vi "nana_4-ZN_O - temp.vi"() -> ()   [LabVIEW 2015]
uses:
  <vilib>/MakerHub/LINX/Public/Peripherals/Digital/Digital Write N Chans.vi
  <vilib>/MakerHub/LINX/Public/Peripherals/Analog/Analog Read 1 Chan.vi
  <vilib>/MakerHub/LINX/Private/Local IO/LinxDigitalWrite.vi
  <vilib>/MakerHub/LINX/Public/Utilities/Check Channel.vi
  <vilib>/MakerHub/LINX/Public/Peripherals/Analog/Analog Read N Chans.vi
  <vilib>/MakerHub/LINX/Private/Local IO/LinxI2cWrite.vi
  <vilib>/MakerHub/LINX/Private/Local IO/LinxAnalogRead.vi
  <vilib>/MakerHub/LINX/Public/Utilities/Open Serial.vi
  <vilib>/MakerHub/LINX/Private/Utilties/Generate Error.vi
  <vilib>/MakerHub/LINX/LMH-LINX.lvlib
panel:
  out "A1":dbl
  out "A2":dbl
  in  "T(V)":dbl
  in  "time post":u32
  in  "number of pulses":i32
  in  "low delay":u32
  in  "peak delay":u32
  out "Ref":dbl(graph)
  in  "LED":refnum<visa-resource-name>="N/A"
  out "3":dbl(graph)
  out "2":dbl(graph)
  out "4":dbl(graph)
  out "1":dbl(graph)
  out "pos":dbl
  in  "milliseconds to wait":u32
  in  "time pre":u32
  in  "Serial Port Analog":refnum<visa-resource-name>="N/A"
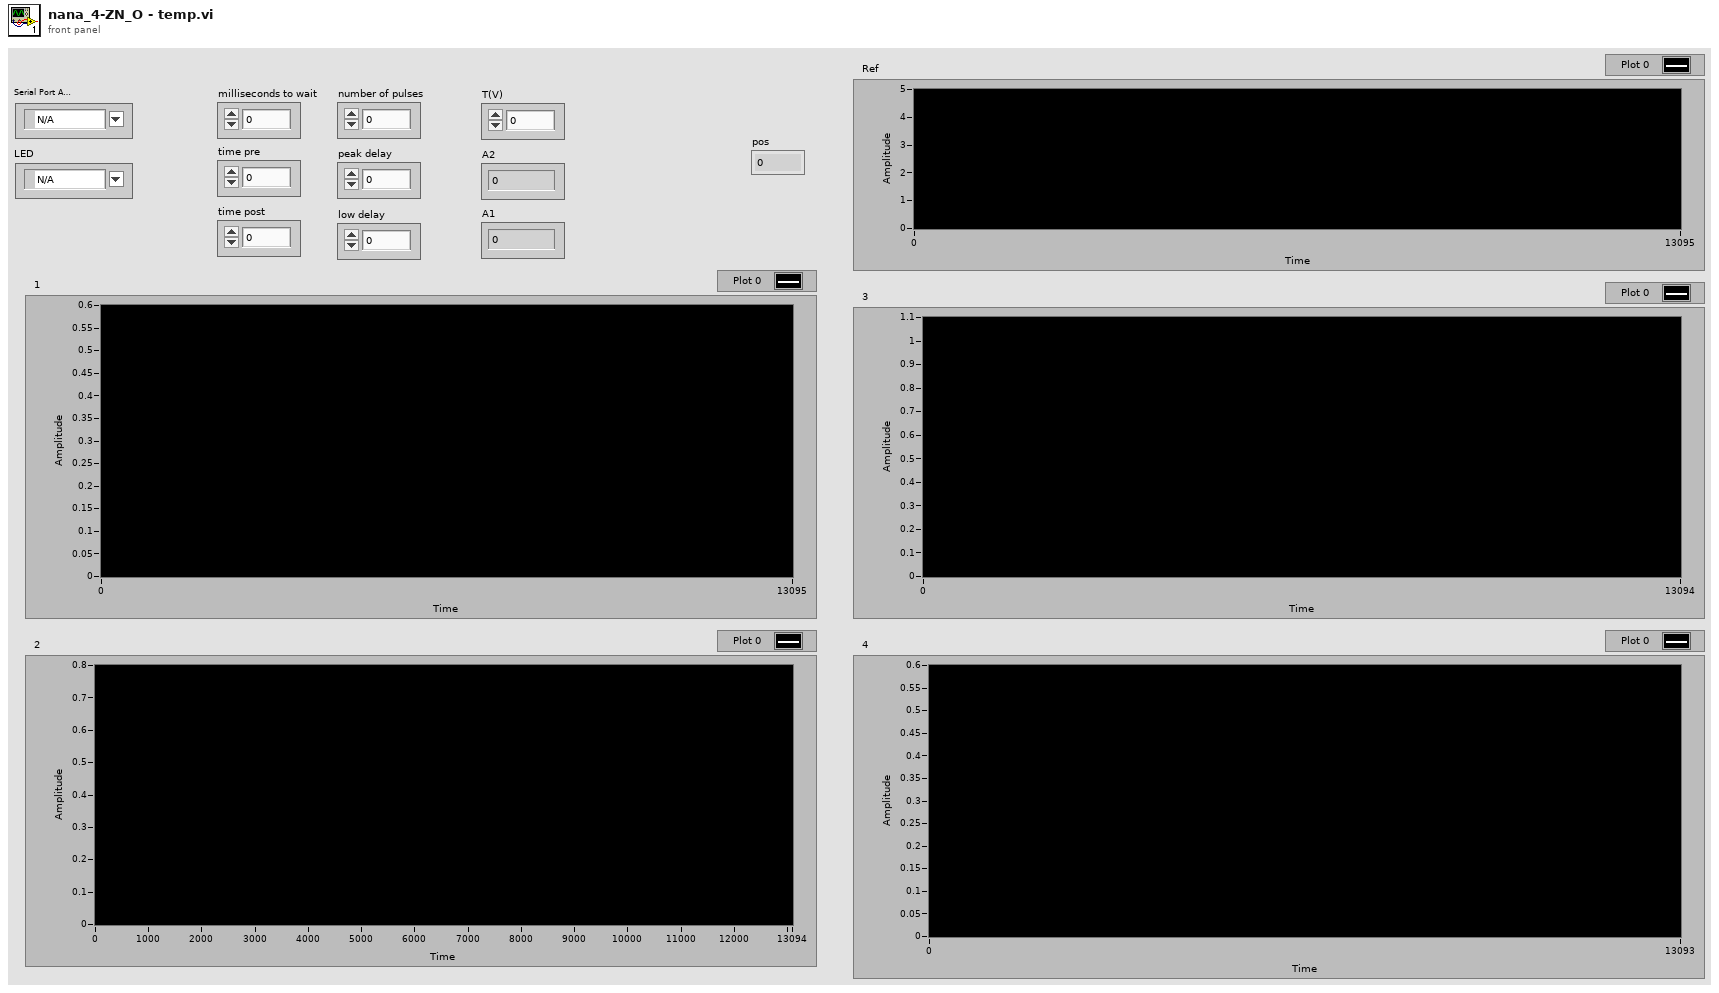
[diagram p1: front panel]
types:
  T1 = typedef "LMH-LINX.lvlib/LINX Ref.ctl" = cluster{"IO":T2, "Interface":T3, "LINX Device Config":T4}
  T2 = typedef "LMH-LINX.lvlib/Platform.ctl" = enum16{"Remote", "Local"}
  T3 = typedef "LMH-LINX.lvlib/Interface.ctl" = enum16{"Serial", "TCP"}
  T4 = typedef "LMH-LINX.lvlib/Device.lvlib/LINX Device Config.ctl" = cluster{"Interface":T3, "COM Port":refnum<visa-resource-name>, "TCP Configuration":T5, "Device Family":u8, "Device ID":u8, "Device Name":string, "TCP Ref":refnum<k5>, "Channels":T6}
  T5 = typedef "LMH-LINX.lvlib/Device.lvlib/TCP Config.ctl" = cluster{"IP Address":string, "Port":u16}
  T6 = typedef "LMH-LINX.lvlib/Channels.ctl" = cluster{"DI":u8[], "DO":u8[], "AI":u8[], "AO":u8[], "PWM":u8[], "QE":u8[], "UART":u8[], "I2C 2":u8[], "SPI":u8[], "CAN":u8[], "Servo":u8[], "AI Ref (V)":dbl, "AI Resolution (Bits)":u8, "AO Ref (V)":dbl, "AO Resolution (Bits)":u8}
  T7 = enum16{"open", "replace", "create", "open or create", "replace or create", "replace or create with confirmation"}
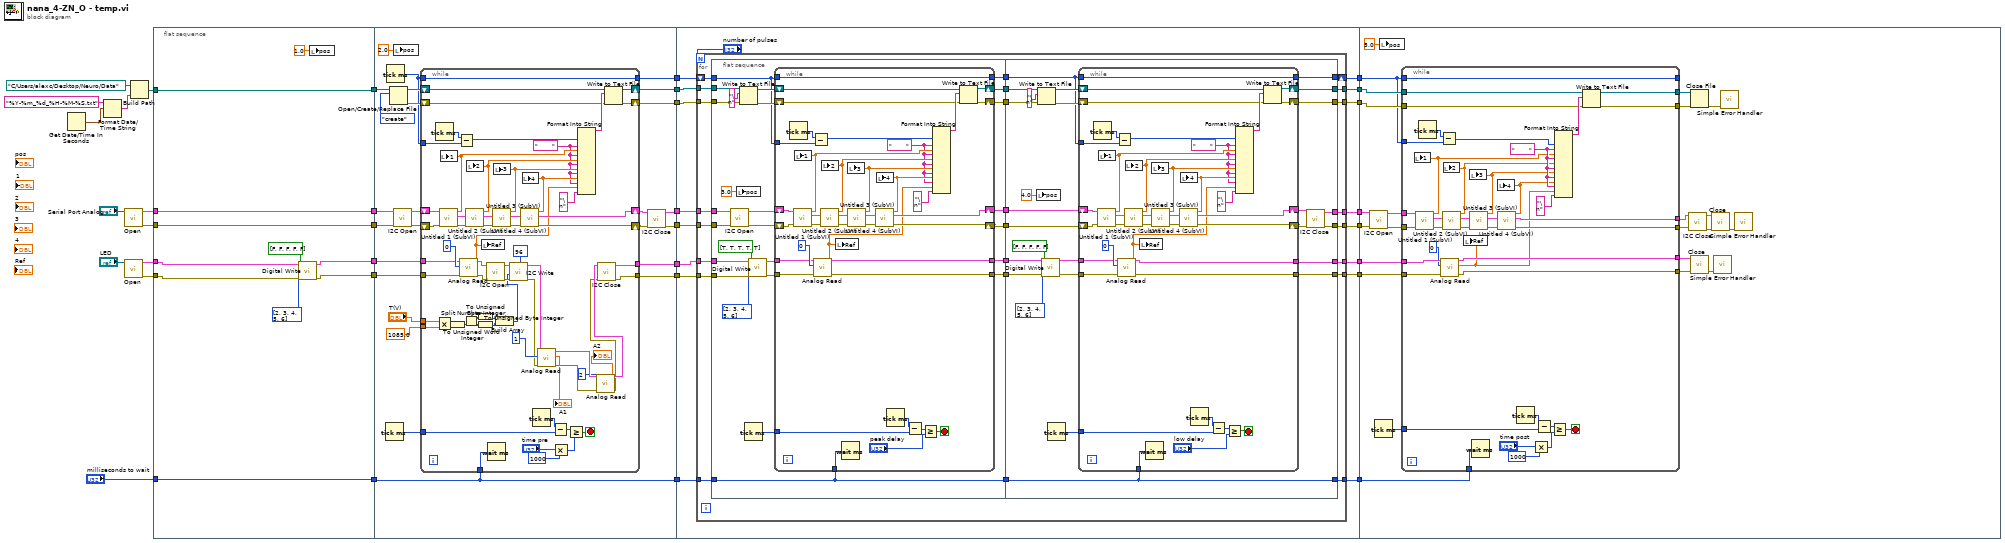
[diagram p0: block diagram]
diagram:
  n1 = Get Date/Time In Seconds() -> (seconds since 1Jan1904=w12:timestamp)
  n2 = Format Date/Time String(time format string (%c)="%Y-%m_%d_%H-%M-%S.txt", seconds (now)=w12) -> (date/time string=w14:string)  [unwired: 1 in]
  n3 = call-poly <vilib>:"Open.vi"("Serial Port"="Serial Port Analog") -> ("Error Out"=w18:errorcluster, "LINX Resource"=w19:T1)  [unwired: 8 in, 1 out]
  n4 = call-poly <vilib>:"Open.vi"("Serial Port"="LED") -> ("Error Out"=w9:errorcluster, "LINX Resource"=w10:T1)  [unwired: 8 in, 1 out]
  n5 = Build Path(base path=path "C:/Users/alexc/Desktop/Neuro/Data", name or relative path=w14) -> (appended path=w11:path)
  n6 = flat-sequence {
    tunnel: [w44] -> w34
    tunnel: [w43] -> w33
    tunnel: [w42] -> w30
    tunnel: [w41] -> w21
    tunnel: w19 -> [w44]
    tunnel: w18 -> [w43]
    tunnel: w11 -> [w42]
    tunnel: w10 -> [w36]
    tunnel: w9 -> [w35]
    tunnel: [w38] -> w8
    tunnel: [w37] -> w7
    tunnel: "milliseconds to wait" -> [w41]
    tunnel: w34 -> [w70]
    tunnel: w33 -> [w69]
    tunnel: [w68] -> w32
    tunnel: [w67] -> w31
    tunnel: w30 -> [w66]
    tunnel: [w62] -> w29
    tunnel: [w61] -> w28
    tunnel: [w59] -> w27
    tunnel: w21 -> [w57]
    tunnel: [w57] -> w20
    tunnel: w8 -> [w51]
    tunnel: w7 -> [w50]
    tunnel: [w49] -> w6
    tunnel: [w48] -> w1
    tunnel: [w139] -> w26
    tunnel: [w138] -> w25
    tunnel: [w142] -> w24
    tunnel: [w141] -> w23
    tunnel: [w140] -> w22
    tunnel: w20 -> [w143]
    tunnel: w27 -> [w147]
    tunnel: w28 -> [w148]
    tunnel: w29 -> [w149]
    tunnel: w31 -> [w145]
    tunnel: w32 -> [w146]
    tunnel: w6 -> [w150]
    tunnel: [w137] -> w4
    tunnel: [w136] -> w3
    tunnel: [w135] -> w2
    tunnel: w1 -> [w134]
    tunnel: w22 -> [w314]
    tunnel: w23 -> [w315]
    tunnel: w24 -> [w301]
    tunnel: w25 -> [w319]
    tunnel: w26 -> [w323]
    tunnel: w4 -> [w318]
    tunnel: w3 -> [w305]
    tunnel: w2 -> [w304]
    frame #0 {
      n7 = call-poly <vilib>:"Digital Write.vi"("Error In"=w35, "Values"=bool[] [FALSE, FALSE, FALSE, FALSE, FALSE], "DO Channels"=u8[] [2, 3, 4, 5, 6], "LINX Resource"=w36) -> ("Error Out"=w37:errorcluster, "LINX Resource"=w38:T1)  [unwired: 6 in]
      n8 = local write "pos"(1.0 ("pos")) -> ()
    }
    frame #1 {
      n9 = Tick Count (ms)() -> (millisecond timer value=w58:u32)
      n10 = Tick Count (ms)() -> (millisecond timer value=w60:u32)
      n11 = Open/Create/Replace File(file path (use dialog)=w66, operation (0:open)=T7."create") -> (refnum out=w64:refnum<file>, error out=w63:errorcluster)  [unwired: 4 in, 1 out]
      n12 = local write "pos"(2.0 ("pos")) -> ()
      n13 = call <vilib>:"I2C Open.vi"("Error In"=w69, "LINX Resource"=w70) -> ("Error Out"=w55:errorcluster, "LINX Resource"=w56:T1)  [unwired: 8 in]
      n14 = while {
        tunnel: w60 -> [w126]
        shift-right: [w122] -> w62
        shift-left: w64 -> [w124]
        shift-right: [w121] -> w61
        shift-left: w63 -> [w123]
        tunnel: [w120] -> w59
        tunnel: w60 -> [w120]
        tunnel: w58 -> [w101]
        tunnel: w57 -> [w104]
        shift-right: [w117] -> w54
        shift-left: w56 -> [w119]
        shift-right: [w116] -> w53
        shift-left: w55 -> [w118]
        tunnel: w51 -> [w106]
        tunnel: w50 -> [w105]
        tunnel: [w72] -> w49
        tunnel: [w71] -> w48
        tunnel: "T(V)" -> [w76]
        tunnel: 1085.0 ("x") -> [w75]
        stop <- w100 stop-if-true
        w110 = "       "
        n15 = Tick Count (ms)() -> (millisecond timer value=w127:u32)
        n16 = Multiply(x=w76, y=w75) -> (x*y=w91:dbl)
        n17 = call "Untitled 1 (SubVI).vi"("error in (no error)"=w118, "LINX Resource in"=w119) -> ("error out"=w132:errorcluster, "LINX Resource out"=w133:T1, "Numeric"=w114:dbl)  [unwired: 7 in]
        n18 = local write "1"(w114) -> ()
        n19 = To Unsigned Word Integer(number=w91) -> (unsigned 16bit integer=w92:u16)
        n20 = Subtract(x=w127, y=w126) -> (x-y=w111:u32)
        n21 = call-poly <vilib>:"Analog Read.vi"("Error In"=w105, "Analog Channel"=u8 0, "LINX Resource"=w106) -> ("Error Out"=w78:errorcluster, "Voltage"=w107:dbl, "LINX Resource"=w79:T1)  [unwired: 5 in, 1 out]
        n22 = Split Number(x=w92) -> (hi(x)=w93:u8, lo(x)=w96:u8)
        n23 = call "Untitled 2 (SubVI).vi"("error in (no error)"=w132, "LINX Resource in"=w133) -> ("error out"=w131:errorcluster, "LINX Resource"=w130:T1, "Numeric"=w113:dbl)  [unwired: 7 in]
        n24 = local write "2"(w113) -> ()
        n25 = To Unsigned Byte Integer(number=w93) -> (unsigned 8bit integer=w95:u8)
        n26 = To Unsigned Byte Integer(number=w96) -> (unsigned 8bit integer=w94:u8)
        n27 = local write "Ref"(w107) -> ()
        n28 = call <vilib>:"I2C Open.vi"("Error In"=w78, "LINX Resource"=w79) -> ("Error Out"=w82:errorcluster, "LINX Resource"=w83:T1)  [unwired: 8 in]
        n29 = Wait (ms)(milliseconds to wait=w104) -> ()  [unwired: 1 out]
        n30 = call "Untitled 3 (SubVI).vi"("error in (no error)"=w131, "LINX Resource in"=w130) -> ("error out"=w128:errorcluster, "LINX Resource out"=w129:T1, "Numeric"=w112:dbl)  [unwired: 7 in]
        n31 = local write "3"(w112) -> ()
        n32 = Build Array(w95, w94) -> (w77:u8[])
        n33 = call <vilib>:"I2C Write.vi"("Error In"=w82, "Data"=w77, "I2C Slave Address (0)"=u8 96, "LINX Resource"=w83) -> ("Error Out"=w80:errorcluster, "LINX Resource"=w81:T1)  [unwired: 6 in]
        n34 = call "Untitled 4 (SubVI).vi"("error in (no error)"=w128, "LINX Resource in"=w129) -> ("error out"=w116:errorcluster, "LINX Resource"=w117:T1, "Numeric"=w115:dbl)  [unwired: 7 in]
        n35 = local write "4"(w115) -> ()
        n36 = Tick Count (ms)() -> (millisecond timer value=w102:u32)
        n37 = call-poly <vilib>:"Analog Read.vi"("Error In"=w80, "Analog Channel"=u8 1, "LINX Resource"=w81) -> ("Error Out"=w88:errorcluster, "Voltage"=→"A1":dbl, "LINX Resource"=w89:T1)  [unwired: 5 in, 1 out]
        n38 = Subtract(x=w102, y=w101) -> (x-y=w103:u32)
        n39 = Multiply(x="time pre", y=u32 1000) -> (x*y=w99:u32)
        n40 = Greater Or Equal?(x=w103, y=w99) -> (x >= y?=w100:bool)
        n41 = Format Into String(w111, w110, w114, w110, w113, w110, w112, w110, w115, w110, w107, "\n") -> (resulting string=w125:string)  [unwired: 3 in, 1 out]
        n42 = call-poly <vilib>:"Analog Read.vi"("Error In"=w88, "Analog Channel"=u8 2, "LINX Resource"=w89) -> ("Error Out"=w73:errorcluster, "Voltage"=→"A2":dbl, "LINX Resource"=w74:T1)  [unwired: 5 in, 1 out]
        n43 = call <vilib>:"I2C Close.vi"("Error In"=w73, "LINX Resource"=w74) -> ("Error Out"=w71:errorcluster, "LINX Resource"=w72:T1)  [unwired: 8 in]
        n44 = Write to Text File(file (use dialog)=w124, text=w125, error in=w123) -> (refnum out=w122:refnum<file>, error out=w121:errorcluster)  [unwired: 1 in, 1 out]
      }
      n45 = call <vilib>:"I2C Close.vi"("Error In"=w53, "LINX Resource"=w54) -> ("Error Out"=w67:errorcluster, "LINX Resource"=w68:T1)  [unwired: 8 in]
    }
    frame #2 {
      n46 = for {
        N: "number of pulses" -> [_]
        tunnel: w150 -> [w174]
        tunnel: w149 -> [w173]
        tunnel: w148 -> [w172]
        shift-right: [w159] -> w142
        shift-left: w147 -> [w169]
        tunnel: w146 -> [w171]
        tunnel: w145 -> [w170]
        tunnel: w143 -> [w161]
        tunnel: [w158] -> w141
        tunnel: [w157] -> w140
        tunnel: [w156] -> w139
        tunnel: [w155] -> w138
        tunnel: [w154] -> w137
        tunnel: [w153] -> w136
        tunnel: [w152] -> w135
        tunnel: w134 -> [w151]
        n47 = flat-sequence {
          tunnel: w174 -> [w195]
          tunnel: w173 -> [w192]
          tunnel: w172 -> [w191]
          tunnel: w171 -> [w184]
          tunnel: w170 -> [w183]
          tunnel: w169 -> [w180]
          tunnel: [w199] -> w168
          tunnel: [w198] -> w167
          tunnel: [w194] -> w166
          tunnel: [w193] -> w165
          tunnel: [w188] -> w164
          tunnel: [w187] -> w163
          tunnel: [w179] -> w162
          tunnel: w161 -> [w176]
          tunnel: [w176] -> w160
          tunnel: w151 -> [w175]
          tunnel: w168 -> [w256]
          tunnel: w167 -> [w255]
          tunnel: w166 -> [w250]
          tunnel: w165 -> [w249]
          tunnel: w164 -> [w252]
          tunnel: w163 -> [w251]
          tunnel: w162 -> [w248]
          tunnel: w160 -> [w240]
          tunnel: [w245] -> w159
          tunnel: [w244] -> w158
          tunnel: [w243] -> w157
          tunnel: [w242] -> w156
          tunnel: [w241] -> w155
          tunnel: [w240] -> w154
          tunnel: [w239] -> w153
          tunnel: [w238] -> w152
          frame #0 {
            n48 = call <vilib>:"I2C Open.vi"("Error In"=w183, "LINX Resource"=w184) -> ("Error Out"=w181:errorcluster, "LINX Resource"=w182:T1)  [unwired: 8 in]
            n49 = local write "pos"(3.0 ("pos")) -> ()
            n50 = Write to Text File(file (use dialog)=w192, text="\n", error in=w191) -> (refnum out=w190:refnum<file>, error out=w189:errorcluster)  [unwired: 1 in, 1 out]
            n51 = Tick Count (ms)() -> (millisecond timer value=w177:u32)
            n52 = call-poly <vilib>:"Digital Write.vi"("Error In"=w175, "Values"=bool[] [TRUE, TRUE, TRUE, TRUE, TRUE], "DO Channels"=u8[] [2, 3, 4, 5, 6], "LINX Resource"=w195) -> ("Error Out"=w186:errorcluster, "LINX Resource"=w185:T1)  [unwired: 6 in]
            n53 = while {
              tunnel: w180 -> [w230]
              shift-right: [w226] -> w194
              shift-left: w190 -> [w228]
              shift-right: [w225] -> w193
              shift-left: w189 -> [w227]
              tunnel: [w224] -> w179
              tunnel: w180 -> [w224]
              tunnel: w177 -> [w201]
              tunnel: w176 -> [w208]
              shift-right: [w221] -> w199
              shift-left: w182 -> [w223]
              shift-right: [w220] -> w198
              shift-left: w181 -> [w222]
              tunnel: w185 -> [w210]
              tunnel: w186 -> [w209]
              tunnel: [w207] -> w188
              tunnel: [w206] -> w187
              stop <- w203 stop-if-true
              w214 = "       "
              n54 = Tick Count (ms)() -> (millisecond timer value=w231:u32)
              n55 = call "Untitled 1 (SubVI).vi"("error in (no error)"=w222, "LINX Resource in"=w223) -> ("error out"=w236:errorcluster, "LINX Resource out"=w237:T1, "Numeric"=w218:dbl)  [unwired: 7 in]
              n56 = local write "1"(w218) -> ()
              n57 = Subtract(x=w231, y=w230) -> (x-y=w215:u32)
              n58 = call-poly <vilib>:"Analog Read.vi"("Error In"=w209, "Analog Channel"=u8 0, "LINX Resource"=w210) -> ("Error Out"=w206:errorcluster, "Voltage"=w211:dbl, "LINX Resource"=w207:T1)  [unwired: 5 in, 1 out]
              n59 = call "Untitled 2 (SubVI).vi"("error in (no error)"=w236, "LINX Resource in"=w237) -> ("error out"=w235:errorcluster, "LINX Resource"=w234:T1, "Numeric"=w217:dbl)  [unwired: 7 in]
              n60 = local write "2"(w217) -> ()
              n61 = local write "Ref"(w211) -> ()
              n62 = Wait (ms)(milliseconds to wait=w208) -> ()  [unwired: 1 out]
              n63 = call "Untitled 3 (SubVI).vi"("error in (no error)"=w235, "LINX Resource in"=w234) -> ("error out"=w232:errorcluster, "LINX Resource out"=w233:T1, "Numeric"=w216:dbl)  [unwired: 7 in]
              n64 = local write "3"(w216) -> ()
              n65 = call "Untitled 4 (SubVI).vi"("error in (no error)"=w232, "LINX Resource in"=w233) -> ("error out"=w220:errorcluster, "LINX Resource"=w221:T1, "Numeric"=w219:dbl)  [unwired: 7 in]
              n66 = local write "4"(w219) -> ()
              n67 = Tick Count (ms)() -> (millisecond timer value=w204:u32)
              n68 = Subtract(x=w204, y=w201) -> (x-y=w205:u32)
              n69 = Greater Or Equal?(x=w205, y="peak delay") -> (x >= y?=w203:bool)
              n70 = Format Into String(w215, w214, w218, w214, w217, w214, w216, w214, w219, w214, w211, "\n") -> (resulting string=w229:string)  [unwired: 3 in, 1 out]
              n71 = Write to Text File(file (use dialog)=w228, text=w229, error in=w227) -> (refnum out=w226:refnum<file>, error out=w225:errorcluster)  [unwired: 1 in, 1 out]
            }
          }
          frame #1 {
            n72 = local write "pos"(4.0 ("pos")) -> ()
            n73 = Write to Text File(file (use dialog)=w250, text="\n", error in=w249) -> (refnum out=w258:refnum<file>, error out=w259:errorcluster)  [unwired: 1 in, 1 out]
            n74 = call-poly <vilib>:"Digital Write.vi"("Error In"=w251, "Values"=bool[] [FALSE, FALSE, FALSE, FALSE, FALSE], "DO Channels"=u8[] [2, 3, 4, 5, 6], "LINX Resource"=w252) -> ("Error Out"=w263:errorcluster, "LINX Resource"=w262:T1)  [unwired: 6 in]
            n75 = Tick Count (ms)() -> (millisecond timer value=w246:u32)
            n76 = while {
              tunnel: w248 -> [w293]
              shift-right: [w289] -> w244
              shift-left: w258 -> [w291]
              shift-right: [w288] -> w243
              shift-left: w259 -> [w290]
              tunnel: [w287] -> w245
              tunnel: w248 -> [w287]
              tunnel: w246 -> [w266]
              tunnel: w240 -> [w271]
              shift-right: [w284] -> w254
              shift-left: w256 -> [w286]
              shift-right: [w283] -> w253
              shift-left: w255 -> [w285]
              tunnel: w262 -> [w273]
              tunnel: w263 -> [w272]
              tunnel: [w270] -> w239
              tunnel: [w269] -> w238
              stop <- w264 stop-if-true
              w277 = "       "
              n77 = Tick Count (ms)() -> (millisecond timer value=w294:u32)
              n78 = call "Untitled 1 (SubVI).vi"("error in (no error)"=w285, "LINX Resource in"=w286) -> ("error out"=w299:errorcluster, "LINX Resource out"=w300:T1, "Numeric"=w281:dbl)  [unwired: 7 in]
              n79 = local write "1"(w281) -> ()
              n80 = Subtract(x=w294, y=w293) -> (x-y=w278:u32)
              n81 = call-poly <vilib>:"Analog Read.vi"("Error In"=w272, "Analog Channel"=u8 0, "LINX Resource"=w273) -> ("Error Out"=w269:errorcluster, "Voltage"=w274:dbl, "LINX Resource"=w270:T1)  [unwired: 5 in, 1 out]
              n82 = call "Untitled 2 (SubVI).vi"("error in (no error)"=w299, "LINX Resource in"=w300) -> ("error out"=w298:errorcluster, "LINX Resource"=w297:T1, "Numeric"=w280:dbl)  [unwired: 7 in]
              n83 = local write "2"(w280) -> ()
              n84 = local write "Ref"(w274) -> ()
              n85 = Wait (ms)(milliseconds to wait=w271) -> ()  [unwired: 1 out]
              n86 = call "Untitled 3 (SubVI).vi"("error in (no error)"=w298, "LINX Resource in"=w297) -> ("error out"=w295:errorcluster, "LINX Resource out"=w296:T1, "Numeric"=w279:dbl)  [unwired: 7 in]
              n87 = local write "3"(w279) -> ()
              n88 = call "Untitled 4 (SubVI).vi"("error in (no error)"=w295, "LINX Resource in"=w296) -> ("error out"=w283:errorcluster, "LINX Resource"=w284:T1, "Numeric"=w282:dbl)  [unwired: 7 in]
              n89 = local write "4"(w282) -> ()
              n90 = Tick Count (ms)() -> (millisecond timer value=w267:u32)
              n91 = Subtract(x=w267, y=w266) -> (x-y=w268:u32)
              n92 = Greater Or Equal?(x=w268, y="low delay") -> (x >= y?=w264:bool)
              n93 = Format Into String(w278, w277, w281, w277, w280, w277, w279, w277, w282, w277, w274, "\n") -> (resulting string=w292:string)  [unwired: 3 in, 1 out]
              n94 = Write to Text File(file (use dialog)=w291, text=w292, error in=w290) -> (refnum out=w289:refnum<file>, error out=w288:errorcluster)  [unwired: 1 in, 1 out]
            }
            n95 = call <vilib>:"I2C Close.vi"("Error In"=w253, "LINX Resource"=w254) -> ("Error Out"=w241:errorcluster, "LINX Resource"=w242:T1)  [unwired: 8 in]
          }
        }
      }
    }
    frame #3 {
      n96 = call <vilib>:"I2C Open.vi"("Error In"=w319, "LINX Resource"=w323) -> ("Error Out"=w316:errorcluster, "LINX Resource"=w317:T1)  [unwired: 8 in]
      n97 = Tick Count (ms)() -> (millisecond timer value=w313:u32)
      n98 = local write "pos"(5.0 ("pos")) -> ()
      n99 = while {
        tunnel: w318 -> [w356]
        tunnel: w317 -> [w355]
        tunnel: w316 -> [w354]
        tunnel: [w348] -> _
        tunnel: w301 -> [w348]
        tunnel: w315 -> [w347]
        tunnel: w314 -> [w346]
        tunnel: w313 -> [w327]
        tunnel: [w345] -> w312
        tunnel: [w344] -> w311
        tunnel: [w343] -> w308
        tunnel: [w342] -> w307
        tunnel: w305 -> [w341]
        tunnel: w304 -> [w340]
        tunnel: [w339] -> w303
        tunnel: [w338] -> w302
        tunnel: w301 -> [w336]
        stop <- w328 stop-if-true
        w358 = "       "
        n100 = call "Untitled 1 (SubVI).vi"("error in (no error)"=w354, "LINX Resource in"=w355) -> ("error out"=w353:errorcluster, "LINX Resource out"=w362:T1, "Numeric"=w350:dbl)  [unwired: 7 in]
        n101 = local write "1"(w350) -> ()
        n102 = Tick Count (ms)() -> (millisecond timer value=w349:u32)
        n103 = Subtract(x=w349, y=w336) -> (x-y=w335:u32)
        n104 = call-poly <vilib>:"Analog Read.vi"("Error In"=w340, "Analog Channel"=u8 0, "LINX Resource"=w341) -> ("Error Out"=w338:errorcluster, "Voltage"=w334:dbl, "LINX Resource"=w339:T1)  [unwired: 5 in, 1 out]
        n105 = call "Untitled 2 (SubVI).vi"("error in (no error)"=w353, "LINX Resource in"=w362) -> ("error out"=w352:errorcluster, "LINX Resource"=w361:T1, "Numeric"=w333:dbl)  [unwired: 7 in]
        n106 = local write "2"(w333) -> ()
        n107 = local write "Ref"(w334) -> ()
        n108 = call "Untitled 3 (SubVI).vi"("error in (no error)"=w352, "LINX Resource in"=w361) -> ("error out"=w351:errorcluster, "LINX Resource out"=w360:T1, "Numeric"=w332:dbl)  [unwired: 7 in]
        n109 = local write "3"(w332) -> ()
        n110 = Wait (ms)(milliseconds to wait=w356) -> ()  [unwired: 1 out]
        n111 = call "Untitled 4 (SubVI).vi"("error in (no error)"=w351, "LINX Resource in"=w360) -> ("error out"=w342:errorcluster, "LINX Resource"=w343:T1, "Numeric"=w331:dbl)  [unwired: 7 in]
        n112 = local write "4"(w331) -> ()
        n113 = Tick Count (ms)() -> (millisecond timer value=w329:u32)
        n114 = Multiply(x="time post", y=u32 1000) -> (x*y=w326:u32)
        n115 = Subtract(x=w329, y=w327) -> (x-y=w330:u32)
        n116 = Greater Or Equal?(x=w330, y=w326) -> (x >= y?=w328:bool)
        n117 = Format Into String(w335, w358, w350, w358, w333, w358, w332, w358, w331, w358, w334, "\n") -> (resulting string=w359:string)  [unwired: 3 in, 1 out]
        n118 = Write to Text File(file (use dialog)=w347, text=w359, error in=w346) -> (refnum out=w345:refnum<file>, error out=w344:errorcluster)  [unwired: 1 in, 1 out]
      }
      n119 = call <vilib>:"I2C Close.vi"("Error In"=w307, "LINX Resource"=w308) -> ("Error Out"=w309:errorcluster, "LINX Resource"=w310:T1)  [unwired: 8 in]
      n120 = Close File(refnum=w312, error in=w311) -> (error out=w322:errorcluster)  [unwired: 1 out]
      n121 = call <vilib>:"Close.vi"("Error In"=w302, "LINX Resource"=w303) -> ("Error Out"=w306:errorcluster)  [unwired: 9 in]
      n122 = call <vilib>:"Close.vi"("Error In"=w309, "LINX Resource"=w310) -> ("Error Out"=w321:errorcluster)  [unwired: 9 in]
      n123 = call <vilib>:"Simple Error Handler.vi"("error in (no error)"=w306) -> ()  [unwired: 4 in, 5 out]
      n124 = call <vilib>:"Simple Error Handler.vi"("error in (no error)"=w322) -> ()  [unwired: 4 in, 5 out]
      n125 = call <vilib>:"Simple Error Handler.vi"("error in (no error)"=w321) -> ()  [unwired: 4 in, 5 out]
    }
  }
